vi "Load File.vi"(8 "error in (no error)":errorcluster, 10 "Path":path, 11 "Excel Interface in":refnum<class "Excel Interface.lvclass">) -> (0 "error out":errorcluster, 2 "cancelled":bool, 3 "Excel Interface out":refnum<class "Excel Interface.lvclass">)   [LabVIEW 2016, in "Excel Interface.lvclass"]
uses:
  Excel Interface.lvclass
  Excel Interface.lvclass/Excel Interface.ctl
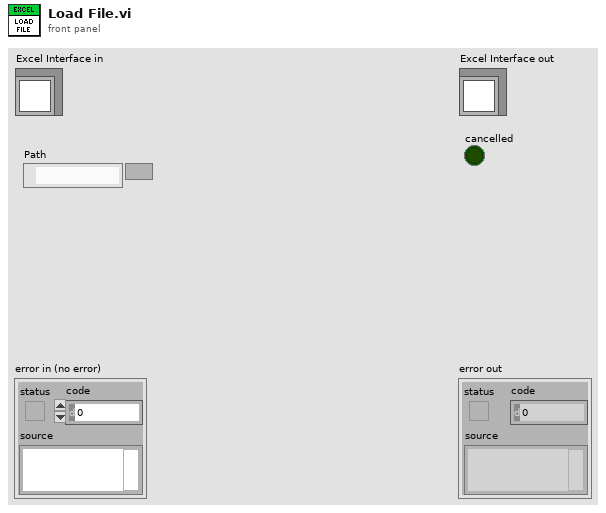
[diagram p1: front panel]
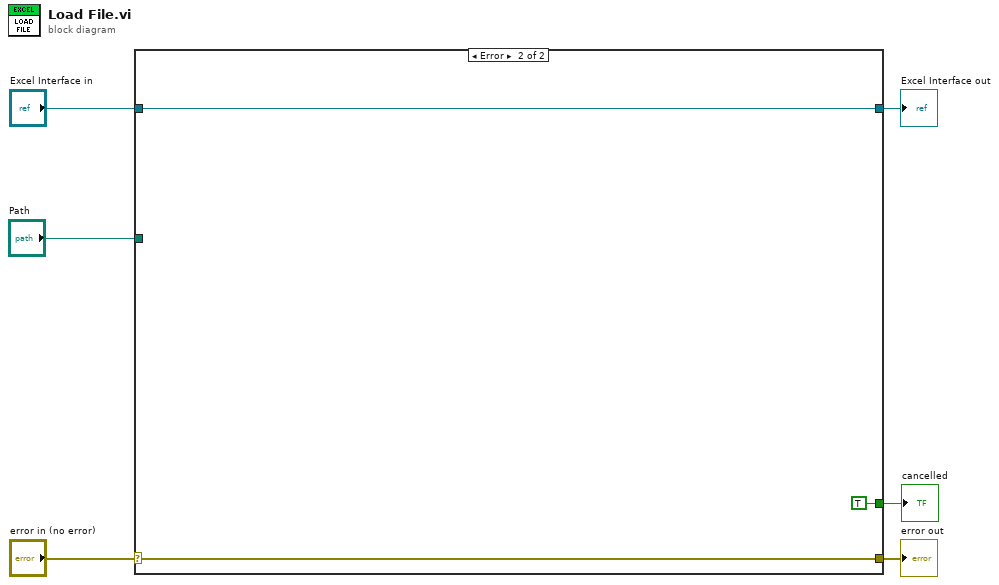
[diagram p0: block diagram]
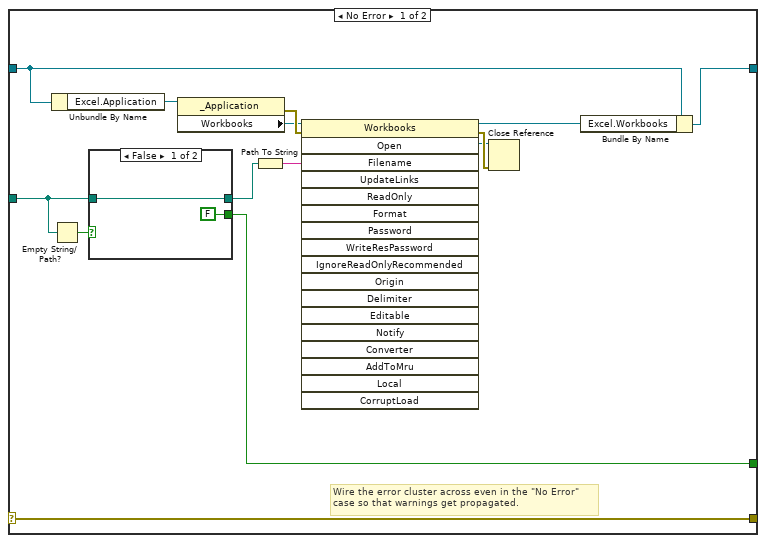
[diagram p2: hidden frame]
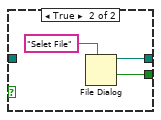
[diagram p3: hidden frame]
diagram:
  n1 = case shown="Error" "error in (no error)" {
    selector: "error in (no error)" -> [w20 w28]
    tunnel: [w20 w28] -> w5
    tunnel: [w8 w27] -> w3
    tunnel: "Excel Interface in" -> [w9 w27]
    tunnel: "Path" -> [w11 _]
    tunnel: [w7 TRUE ("cancelled")] -> w1
    frame No Error {
      # "Wire the error cluster across even in the \"No Error\"\ncase so that warnings get propagated."
      n2 = Unbundle By Name(w9) -> ("Excel.Application"=w13:refnum<k7>)
      n3 = Empty String/Path?(string/path=w11) -> (empty?=w12:bool)
      n4 = case shown="False" w12 {
        tunnel: [w22 w24] -> w15
        tunnel: w11 -> [w22 _]
        tunnel: [FALSE ("cancelled") w23] -> w7
        frame False {
        }
        frame True {
          n5 = File Dialog(7:"Selet File" ("prompt")) -> (1:w23:bool, 3:w24:path)  [unwired: 6 in, 2 out]
        }
      }
      n6 = property class="_Application"(reference=w13) -> (error out=w19:errorcluster, "Workbooks"=w16:refnum<k7>)  [unwired: 1 in, 1 out]
      n7 = Path To String(path=w15) -> (string=w14:string)
      n8 = invoke class="Workbooks" method="Open"(reference=w16, error in=w19, "Filename"=w14) -> (reference out=w10:refnum<k7>, error out=w18:errorcluster, "Open"=w17:refnum<k7>)  [unwired: 15 in, 15 out]
      n9 = Close Reference(reference=w17, error in (no error)=w18) -> ()  [unwired: 1 out]
      n10 = Bundle By Name(cluster=w9, "Excel.Workbooks"=w10) -> (w8:refnum<class "Excel Interface.lvclass">)
    }
    frame Error {
    }
  }
  "error out" <- w5
  "Excel Interface out" <- w3
  "cancelled" <- w1
